vi "Auto Probe Sense Value.vi"(8 "error in (no error)":errorcluster {"code" format="%.0x"}, 10 "Channel (\"CH1\")":string(combo)="CH1", 11 "VISA Resource Name":refnum<visa-resource-name>) -> (0 "error out":errorcluster {"code" format="%.0x"}, 2 "auto probe sense value":dbl caption="Auto Probe Sense Value" format="%.2p", 3 "VISA Resource Name Out":refnum<visa-resource-name>)   [LabVIEW 2010, in "Tektronix TDS 3000 Series.lvlib"]
doc: "The VI returns the probe attenuation value the oscilloscope senses."
uses:
  <instrlib>/Tektronix TDS 3000 Series/Tektronix TDS 3000 Series.lvlib
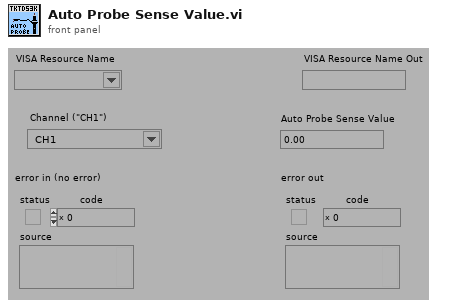
[diagram p1: front panel]
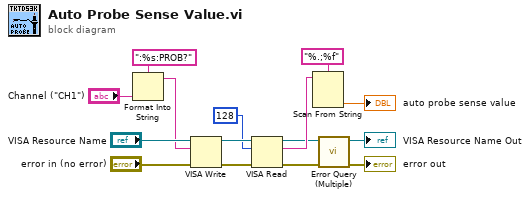
[diagram p0: block diagram]
diagram:
  n1 = Format Into String(format string=":%s:PROB?", "Channel (\"CH1\")") -> (resulting string=w9:string)  [unwired: 2 in, 1 out]
  n2 = VISA Write(VISA resource name="VISA Resource Name", write buffer=w9, error in (no error)="error in (no error)") -> (VISA resource name out=w15:refnum<visa-resource-name>, error out=w14:errorcluster)  [unwired: 1 out]
  n3 = VISA Read(VISA resource name=w15, byte count=u32 128, error in (no error)=w14) -> (VISA resource name out=w4:refnum<visa-resource-name>, read buffer=w6:string, error out=w1:errorcluster)  [unwired: 1 out]
  n4 = Scan From String(format string="%.;%f", input string=w6) -> (output 1=→"auto probe sense value":dbl)  [unwired: 3 in, 3 out]
  n5 = call <instrlib>:"Error Query (Multiple).vi"("error in (no error)"=w1, "VISA Resource Name"=w4) -> ("error out"=→"error out":errorcluster, "VISA Resource Name Out"=→"VISA Resource Name Out":refnum<visa-resource-name>)  [unwired: 6 in, 2 out]
